vi "Do.vi"(8 "error in":errorcluster, 10 "Actor in":refnum<class "Actor.lvclass">, 11 "Set Modulation MSG":refnum<class "Set Modulation MSG.lvclass">) -> (0 "error out":errorcluster, 2 "Actor out":refnum<class "Actor.lvclass">)   [LabVIEW 2014, in "ePAS Library.lvlib" / "Set Modulation MSG.lvclass"]
doc: "(<B>Filename</B>: Actor Framework.lvlib:Message.lvclass:Do.vi)\n\nDefines what a message does when it is received by an actor. Generally, a message instructs an actor to invoke one of its methods. By default, this method does nothing. A child class must override it to define behavior. Create a child class by using the Actor Framework Message Maker dialog box."
uses:
  Set Modulation MSG.lvclass
  <vilib>/ActorFramework/Actor/Actor.lvclass
  Set Modulation MSG.lvclass/Set Modulation MSG.ctl
  Instr Actor.lvclass
  SuperActor/SuperActor.lvclass/SuperActor.ctl
  PAS/Commands/Change Laser Modulation/Change Laser Modulation.lvclass
  PAS/Commands/Change Laser Modulation/Change Laser Modulation.lvclass/Change Laser Modulation.ctl
  PAS/Commands/Change Laser Modulation/Write Modulation.vi
  SuperActor/Read CVT Session.vi
  Accessors/Read CMD.vi
  reusable/Command/Command.lvclass
  <userlib>/_Session Fwk/Session - Root.lvclass
  reusable/Session APIs/CVT/CVT.lvclass
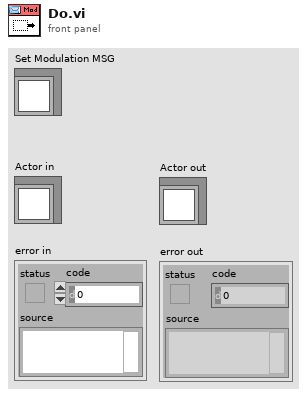
[diagram p1: front panel]
types:
  T1 = typedef "Session - Root.lvclass/Session Handle.ctl" = refnum<data-value>
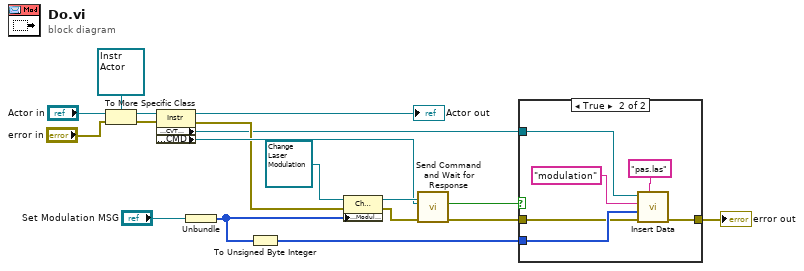
[diagram p0: block diagram]
diagram:
  n1 = To More Specific Class(target class=refnum<class "Instr Actor.lvclass"> refnum ("Instrument Lib:Instr"), reference="Actor in", error in="error in") -> (specific class reference=w11:refnum<class "Instr Actor.lvclass">, error out=w10:errorcluster)
  n2 = property class="Instr"(reference=w11, error in=w10) -> (reference out=→"Actor out":refnum<class "Instr Actor.lvclass">, error out=w7:errorcluster, "Accessors:CVT Session"=w3:T1, "Accessors:CMD"=w9:refnum<queue>)
  n3 = Unbundle("Set Modulation MSG") -> (w12:enum8{"Sine", "Square"}[])
  n4 = To Unsigned Byte Integer(number=w12) -> (unsigned 8bit integer=w4:u8[])
  n5 = property class="Change Laser Modulation.lvclass"(reference=refnum<class "Change Laser Modulation.lvclass"> refnum ("Change Laser Modulation.lvclass"), error in=w7, "Accessors:Modulation"=w12) -> (reference out=w13:refnum<class "Change Laser Modulation.lvclass">, error out=w6:errorcluster)
  n6 = call "Send Command and Wait for Response.vi"("error in"=w6, "cmd queue"=w9, "CMD in"=w13) -> ("error out"=w5:errorcluster, "cmd good?"=w1:bool)  [unwired: 6 in, 1 out]
  n7 = case shown="True" w1 {
    tunnel: w4 -> [_ w22]
    tunnel: w5 -> [w19 w21]
    tunnel: [w19 w20] -> w2
    tunnel: w3 -> [_ w25]
    frame False {
    }
    frame True {
      n8 = call "Insert Data.vi"("Group"="pas.las", "error in"=w21, "Data"=w22, "tag"="modulation" ("Key"), "CVT Session In"=w25) -> ("error out"=w20:errorcluster)  [unwired: 5 in, 1 out]
    }
  }
  "error out" <- w2
